vi "AH2700Monitor.vi"() -> ()   [LabVIEW 2019]
uses:
  Utility/Monitor Communication/AH2700/AH2700-Cluster.ctl
  Instrument_Setup.vi
  Global/Global Variables/Data_Display_global.vi
  Global/Global Variables/global.vi
  Equipment/Capacity_Bridge_AH2700A/Andeen-Hagerling 2700/Andeen-Hagerling 2700.lvlib
panel:
  out "Error Massege":string
  in  "Total 2":i32 min=0 max=99999999
  in  "Interval 2":dbl min=0.0 max=99999999.0 step=0.1 format="%#_10f"
  out "AH 2700-Cluster":T1={"Units Display"=1, "Sample Switch"=0, "Frequency"=0.0, "V excitation"=0.0, "Capacity Graphic"=[], "Loss Graphic"=[], "Capacity"=0.0, "Loss"=0.0, "Update AH2500"=FALSE, "Bias "=0.0, " AVerage"=0.0} {"V excitation" format="%#_6f"; "Units Display" items=["nanosiemens"=1, "dissipation factor"=2, "kilohms"=3, "gigohms"=4, "loss vector (jpF)"=5]}
  in  "stop":bool
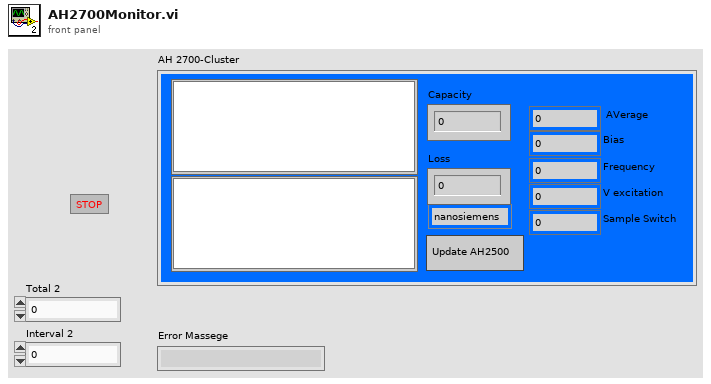
[diagram p1: front panel]
types:
  T1 = typedef "AH2700-Cluster.ctl" = cluster{"Units Display":i32, "Sample Switch":i32, "Frequency":dbl, "V excitation":dbl, "Capacity Graphic":dbl[][], "Loss Graphic":dbl[][], "Capacity":dbl, "Loss":dbl, "Update AH2500":bool, "Bias ":dbl, " AVerage":dbl}
  T2 = cluster{"AVerage":dbl, "Bias":dbl, "V excitation":dbl, "AH Frequency":dbl}
  T3 = cluster{"Baud Rate":u32, "Parity":u16, "Data Bits":u16, "Stop Bits":u16}
  T4 = typedef "AH2700-Control.ctl" = cluster{"Update AH2500":bool}
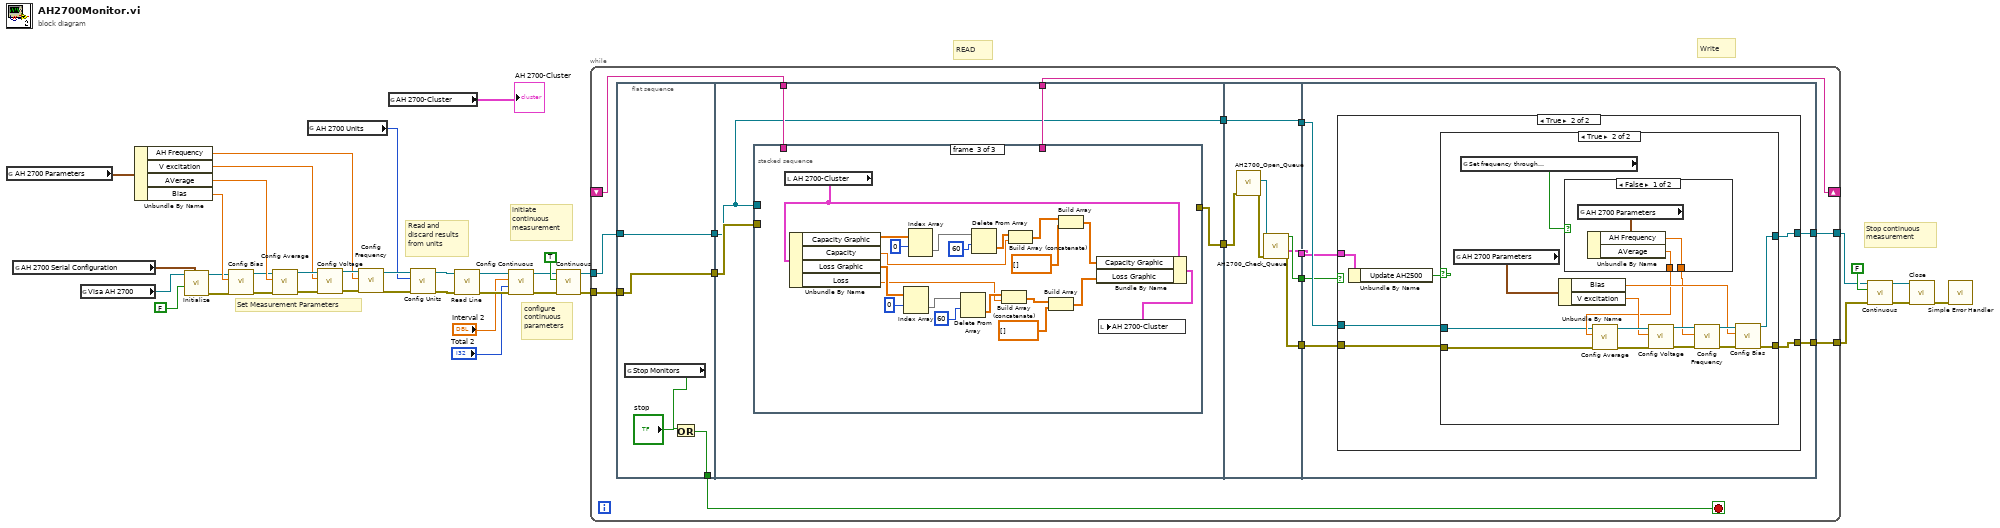
[diagram p0: block diagram]
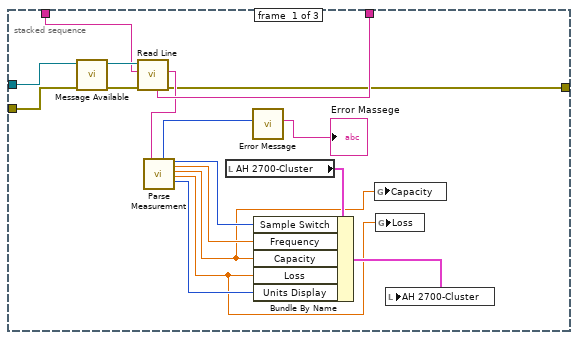
[diagram p2: hidden frame]
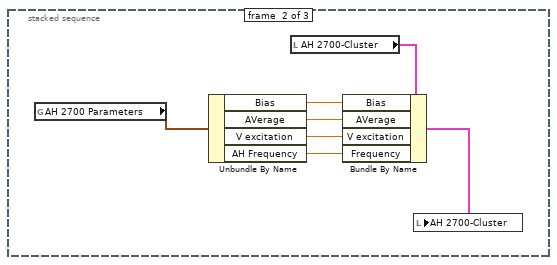
[diagram p3: hidden frame]
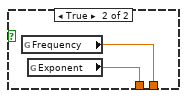
[diagram p6: hidden frame]
diagram:
  # "Stop continuous\nmeasurement"
  # "Write"
  # "READ"
  # "configure\ncontinuous\nparameters"
  # "initiate\ncontinuous\nmeasurement"
  # "Set Measurement Parameters"
  # "Read and\ndiscard results\nfrom units"
  n1 = global read "Instrument_Setup.vi" "AH 2700 Parameters"() -> (w16:T2)
  n2 = global read "Instrument_Setup.vi" "AH 2700 Serial Configuration"() -> (w13:T3)
  n3 = global read "Instrument_Setup.vi" "Visa AH 2700"() -> (w20:refnum<visa-resource-name>)
  n4 = Unbundle By Name(w16) -> ("AH Frequency"=w12:dbl, "V excitation"=w15:dbl, "AVerage"=w14:dbl, "Bias"=w9:dbl)
  n5 = call "Initialize.vi"("Serial Configuration"=w13, "Reset (True)"=FALSE, "VISA resource name"=w20) -> ("error out"=w7:errorcluster, "VISA resource name out"=w8:refnum<visa-resource-name>)  [unwired: 7 in]
  n6 = call "Config Bias.vi"("error in"=w7, "Bias (Off)"=w9, "VISA resource name"=w8) -> ("error out"=w10:errorcluster, "VISA resource name out"=w11:refnum<visa-resource-name>)  [unwired: 7 in]
  n7 = call "Config Average.vi"("error in"=w10, "Average Exponent (4)"=w14, "VISA resource name"=w11) -> ("error out"=w33:errorcluster, "VISA resource name out"=w36:refnum<visa-resource-name>)  [unwired: 7 in]
  n8 = global read "Instrument_Setup.vi" "AH 2700 Units"() -> (w21:i32)
  n9 = call "Config Voltage.vi"("error in"=w33, "Voltage (15 V)"=w15, "VISA resource name"=w36) -> ("error out"=w32:errorcluster, "VISA resource name out"=w35:refnum<visa-resource-name>)  [unwired: 7 in]
  n10 = call "Config Frequency.vi"("error in"=w32, "Frequency (1000 Hz)"=w12, "VISA resource name"=w35) -> ("error out"=w31:errorcluster, "VISA resource name out"=w34:refnum<visa-resource-name>)  [unwired: 7 in]
  n11 = global read "Data_Display_global.vi" "AH 2700-Cluster"() -> (→"AH 2700-Cluster":T1)
  n12 = call "Config Units.vi"("error in"=w31, "Units (nS)"=w21, "VISA resource name"=w34) -> ("error out"=w29:errorcluster, "VISA resource name out"=w30:refnum<visa-resource-name>)  [unwired: 7 in]
  n13 = call "Read Line.vi"("error in"=w29, "VISA resource name"=w30) -> ("error out"=w25:errorcluster, "VISA resource name out"=w27:refnum<visa-resource-name>)  [unwired: 5 in, 3 out]
  n14 = call "Config Continuous.vi"("error in"=w25, "Total (0)"="Total 2", "Interval (0)"="Interval 2", "VISA resource name"=w27) -> ("error out"=w24:errorcluster, "VISA resource name out"=w26:refnum<visa-resource-name>)  [unwired: 6 in]
  n15 = call "Continuous.vi"("error in"=w24, "Continuous Measurement (true)"=TRUE ("On (true)"), "VISA resource name"=w26) -> ("error out"=w18:errorcluster, "VISA resource name out"=w19:refnum<visa-resource-name>)  [unwired: 7 in]
  n16 = while {
    tunnel: w19 -> [w50]
    tunnel: w18 -> [w48]
    shift-right: [w47] -> _
    shift-left: _ -> [w46]
    tunnel: [w42] -> w2
    tunnel: [w41] -> w1
    stop <- w52 stop-if-true
    n17 = flat-sequence {
      tunnel: [w55] -> w52
      tunnel: [w54] -> w51
      tunnel: w50 -> [w54]
      tunnel: [w53] -> w49
      tunnel: w48 -> [w53]
      tunnel: w51 -> [w58]
      tunnel: w49 -> [w62]
      tunnel: [w61] -> w47
      tunnel: w46 -> [w60]
      tunnel: [w59] -> w45
      tunnel: [w58] -> w43
      tunnel: w45 -> [w112]
      tunnel: [w113] -> w44
      tunnel: w43 -> [w113]
      tunnel: [w109] -> w40
      tunnel: [w108] -> w39
      tunnel: [w107] -> w38
      tunnel: w44 -> [w119]
      tunnel: [w118] -> w42
      tunnel: [w117] -> w41
      tunnel: w40 -> [w116]
      tunnel: w39 -> [w115]
      tunnel: w38 -> [w114]
      frame #0 {
        n18 = global read "Data_Display_global.vi" "Stop Monitors"() -> (w57:bool)
        n19 = Or(x=w57, y="stop") -> (x .or. y?=w55:bool)
      }
      frame #1 {
        n20 = stacked-sequence {
          tunnel: w58 -> [w79 _ _]
          tunnel: w62 -> [w78 _ _]
          tunnel: [w75 _ _] -> w61
          tunnel: w60 -> [w74 _ _]
          tunnel: [w65 _ _] -> w59
          frame #0 {
            n21 = call "Message Available.vi"("error in"=w78, "VISA resource name"=w79) -> ("error out"=w76:errorcluster, "VISA resource name out"=w77:refnum<visa-resource-name>)  [unwired: 7 in, 1 out]
            n22 = call "Read Line.vi"("error in"=w76, "Previous"=w74, "VISA resource name"=w77) -> ("error out"=w65:errorcluster, "Message"=w73:string, "Remaining"=w75:string)  [unwired: 4 in, 2 out]
            n23 = call "Parse Measurement.vi"("Measurement Line"=w73) -> ("Error Code"=w72:i32, "Sample"=w69:i32, "Frequency"=w68:dbl, "Capacitance"=w64:dbl, "Loss"=w63:dbl, "Units"=w67:i32)  [unwired: 10 in, 3 out]
            n24 = local read "AH 2700-Cluster"() -> (w71:T1)
            n25 = call "Error Message.vi"("Error Code"=w72) -> ("Error Message"=→"Error Massege":string)  [unwired: 10 in]
            n26 = Bundle By Name(cluster=w71, "Sample Switch"=w69, "Frequency"=w68, "Capacity"=w64, "Loss"=w63, "Units Display"=w67) -> (w70:T1)
            n27 = global write "Data_Display_global.vi" "Capacity"(w64) -> ()
            n28 = global write "Data_Display_global.vi" "Loss"(w63) -> ()
            n29 = local write "AH 2700-Cluster"(w70) -> ()
          }
          frame #1 {
            n30 = global read "Instrument_Setup.vi" "AH 2700 Parameters"() -> (w84:T2)
            n31 = Unbundle By Name(w84) -> ("Bias"=w83:dbl, "AVerage"=w82:dbl, "V excitation"=w81:dbl, "AH Frequency"=w80:dbl)
            n32 = local read "AH 2700-Cluster"() -> (w86:T1)
            n33 = Bundle By Name(cluster=w86, "Bias"=w83, "AVerage"=w82, "V excitation"=w81, "Frequency"=w80) -> (w85:T1)
            n34 = local write "AH 2700-Cluster"(w85) -> ()
          }
          frame #2 {
            n35 = local read "AH 2700-Cluster"() -> (w94:T1)
            n36 = Unbundle By Name(w94) -> ("Capacity Graphic"=w106:dbl[][], "Capacity"=w97:dbl, "Loss Graphic"=w104:dbl[][], "Loss"=w95:dbl)
            n37 = Index Array(array=w104, index (row)=0) -> (element=w99:dbl[])  [unwired: 1 in]
            n38 = Index Array(array=w106, index (row)=0) -> (element=w102:dbl[])  [unwired: 1 in]
            n39 = Delete From Array(array=w99, length=60) -> (deleted portion=w96:dbl[])  [unwired: 1 in, 1 out]
            n40 = Delete From Array(array=w102, length=60) -> (deleted portion=w98:dbl[])  [unwired: 1 in, 1 out]
            n41 = Build Array (concatenate)(w96, w95) -> (w89:dbl[])
            n42 = Build Array (concatenate)(w98, w97) -> (w92:dbl[])
            n43 = Build Array(w89, dbl[] []) -> (w87:dbl[][])
            n44 = Build Array(w92, dbl[] []) -> (w90:dbl[][])
            n45 = Bundle By Name(cluster=w94, "Capacity Graphic"=w90, "Loss Graphic"=w87) -> (w93:T1)
            n46 = local write "AH 2700-Cluster"(w93) -> ()
          }
        }
      }
      frame #2 {
        n47 = call "AH2700_Open_Queue.vi"("error in (no error)"=w112) -> ("error out"=w110:errorcluster, "queue out"=w111:refnum<queue>)  [unwired: 9 in]
        n48 = call "AH2700_Check_Queue.vi"("error in (no error)"=w110, "Queue"=w111) -> ("error out"=w108:errorcluster, "AH2700-Control"=w107:T4, "New Entries?"=w109:bool)  [unwired: 6 in]
      }
      frame #3 {
        n49 = case shown="True" w116 {
          tunnel: w119 -> [w121 w122]
          tunnel: [w121 w127] -> w118
          tunnel: [w120 w126] -> w117
          tunnel: w115 -> [w120 w125]
          tunnel: w114 -> [_ w124]
          frame False {
          }
          frame True {
            n50 = Unbundle By Name(w124) -> ("Update AH2500"=w123:bool)
            n51 = case shown="True" w123 {
              tunnel: w122 -> [w129 w133]
              tunnel: [w129 w132] -> w127
              tunnel: [w128 w131] -> w126
              tunnel: w125 -> [w128 w130]
              frame False {
              }
              frame True {
                n52 = global read "Instrument_Setup.vi" "AH 2700 Parameters"() -> (w140:T2)
                n53 = global read "Instrument_Setup.vi" "Set frequency through\ncommand file"() -> (w145:bool)
                n54 = Unbundle By Name(w140) -> ("Bias"=w136:dbl, "V excitation"=w139:dbl)
                n55 = case shown="False" w145 {
                  tunnel: [w146 w150] -> w135
                  tunnel: [w147 w149] -> w134
                  frame False {
                    n56 = global read "Instrument_Setup.vi" "AH 2700 Parameters"() -> (w148:T2)
                    n57 = Unbundle By Name(w148) -> ("AH Frequency"=w146:dbl, "AVerage"=w147:dbl)
                  }
                  frame True {
                    n58 = global read "global.vi" "Frequency"() -> (w150:dbl)
                    n59 = global read "global.vi" "Exponent"() -> (w149:dbl)
                  }
                }
                n60 = call "Config Average.vi"("error in"=w130, "Average Exponent (4)"=w134, "VISA resource name"=w133) -> ("error out"=w143:errorcluster, "VISA resource name out"=w144:refnum<visa-resource-name>)  [unwired: 7 in]
                n61 = call "Config Voltage.vi"("error in"=w143, "Voltage (15 V)"=w139, "VISA resource name"=w144) -> ("error out"=w141:errorcluster, "VISA resource name out"=w142:refnum<visa-resource-name>)  [unwired: 7 in]
                n62 = call "Config Frequency.vi"("error in"=w141, "Frequency (1000 Hz)"=w135, "VISA resource name"=w142) -> ("error out"=w137:errorcluster, "VISA resource name out"=w138:refnum<visa-resource-name>)  [unwired: 7 in]
                n63 = call "Config Bias.vi"("error in"=w137, "Bias (Off)"=w136, "VISA resource name"=w138) -> ("error out"=w131:errorcluster, "VISA resource name out"=w132:refnum<visa-resource-name>)  [unwired: 7 in]
              }
            }
          }
        }
      }
    }
  }
  n64 = call "Continuous.vi"("error in"=w1, "Continuous Measurement (true)"=FALSE ("On (true)"), "VISA resource name"=w2) -> ("error out"=w6:errorcluster, "VISA resource name out"=w5:refnum<visa-resource-name>)  [unwired: 7 in]
  n65 = call "Close.vi"("error in (no error)"=w6, "VISA resource name"=w5) -> ("error out"=w3:errorcluster)  [unwired: 9 in]
  n66 = call <vilib>:"Simple Error Handler.vi"("error in (no error)"=w3) -> ()  [unwired: 4 in, 5 out]
